vi "sum_gist1m1.vi"(3 "Y":i16[](array[numeric]), 5 "hist in":cluster{i16[], i32[]}) -> (1 "hist":cluster{i16[], i32[]})   [LabVIEW 2010]
panel:
  # "Сложение гистограммы с массивом"
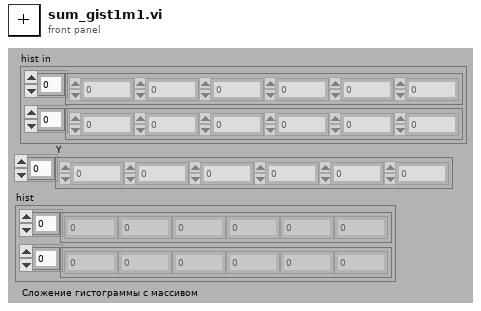
[diagram p1: front panel]
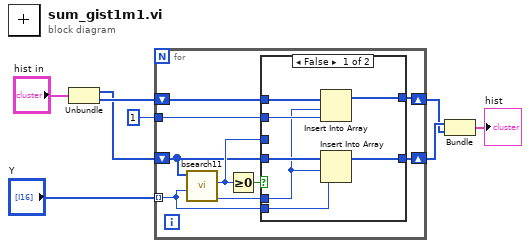
[diagram p0: block diagram]
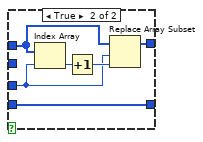
[diagram p2: hidden frame]
diagram:
  n1 = Unbundle("hist in") -> (w1:i16[], w2:i32[])
  n2 = for {
    tunnel: "Y" -> [w10] mode=indexing
    shift-right: [w17] -> w6
    shift-left: w1 -> [w11]
    shift-right: [w15] -> w5
    shift-left: w2 -> [w14]
    tunnel: 1 ("dimension size") -> [w13]
    n3 = call "bsearch11.vi"("val"=w10, "Array"=w11) -> ("a"=w9:i32, "idx"=w12:i32)  [unwired: 4 in]
    n4 = Greater Or Equal To 0?(x=w12) -> (x >= 0?=w16:bool)
    n5 = case shown="False" w16 {
      tunnel: w11 -> [w24 w30]
      tunnel: [w23 w30] -> w17
      tunnel: w10 -> [w22 _]
      tunnel: [w21 w26] -> w15
      tunnel: w14 -> [w20 w27]
      tunnel: w12 -> [_ w25]
      tunnel: w13 -> [w19 _]
      tunnel: w9 -> [w18 _]
      frame False {
        n6 = Insert Into Array(array=w20, index=w18, new element=w19) -> (w21:i32[])
        n7 = Insert Into Array(array=w24, index=w18, new element=w22) -> (w23:i16[])
      }
      frame True {
        n8 = Index Array(array=w27, index=w25) -> (element=w29:i32)
        n9 = Increment(x=w29) -> (x+1=w28:i32)
        n10 = Replace Array Subset(array=w27, new element=w28, index=w25) -> (w26:i32[])
      }
    }
  }
  n11 = Bundle(w6, w5) -> (→"hist":cluster{i16[], i32[]})  [unwired: 1 in]
